vi "rs3 set device option2.vi"(8 "error in (no error)":errorcluster, 9 "value":sgl, 10 "RS Option":u16(ring) items=["    RS2_OPTION_BACKLIGHT_COMPENSATION                     , /**< Enable / disable color backlight compensation*/", "    RS2_OPTION_BRIGHTNESS                                 , /**< Color image brightness*/", "    RS2_OPTION_CONTRAST                                   , /**< Color image contrast*/", "    RS2_OPTION_EXPOSURE                                   , /**< Controls exposure time of color camera. Setting any value will disable auto exposure*/", "    RS2_OPTION_GAIN                                       , /**< Color image gain*/", "    RS2_OPTION_GAMMA                                      , /**< Color image gamma setting*/", "    RS2_OPTION_HUE                                        , /**< Color image hue*/", "    RS2_OPTION_SATURATION                                 , /**< Color image saturation setting*/", "    RS2_OPTION_SHARPNESS                                  , /**< Color image sharpness setting*/", "    RS2_OPTION_WHITE_BALANCE                              , /**< Controls white balance of color image. Setting any value will disable auto white balance*/", "    RS2_OPTION_ENABLE_AUTO_EXPOSURE                       , /**< Enable / disable color image auto-exposure*/", "    RS2_OPTION_ENABLE_AUTO_WHITE_BALANCE                  , /**< Enable / disable color image auto-white-balance*/", "    RS2_OPTION_VISUAL_PRESET                              , /**< Provide access to several recommend sets of option presets for the depth camera */", "    RS2_OPTION_LASER_POWER                                , /**< Power of the F200 / SR300 projector, with 0 meaning projector off*/", "    RS2_OPTION_ACCURACY                                   , /**< Set the number of patterns projected per frame. The higher the accuracy value the more patterns projected. Increasing the number of patterns help to achieve better accuracy. Note that this c", "    RS2_OPTION_MOTION_RANGE                               , /**< Motion vs. Range trade-off, with lower values allowing for better motion sensitivity and higher values allowing for better depth range*/", "    RS2_OPTION_FILTER_OPTION                              , /**< Set the filter to apply to each depth frame. Each one of the filter is optimized per the application requirements*/", "    RS2_OPTION_CONFIDENCE_THRESHOLD                       , /**< The confidence level threshold used by the Depth algorithm pipe to set whether a pixel will get a valid range or will be marked with invalid range*/", "    RS2_OPTION_EMITTER_ENABLED                            , /**< Laser Emitter enabled */", "    RS2_OPTION_FRAMES_QUEUE_SIZE                          , /**< Number of frames the user is allowed to keep per stream. Trying to hold-on to more frames will cause frame-drops.*/", "    RS2_OPTION_TOTAL_FRAME_DROPS                          , /**< Total number of detected frame drops from all streams */", "    RS2_OPTION_AUTO_EXPOSURE_MODE                         , /**< Auto-Exposure modes: Static, Anti-Flicker and Hybrid */", "    RS2_OPTION_AUTO_EXPOSURE_ANTIFLICKER_RATE             , /**< Auto-Exposure anti-flicker rate, can be 50 or 60 Hz */", "    RS2_OPTION_ASIC_TEMPERATURE                           , /**< Current Asic Temperature */", "    RS2_OPTION_ERROR_POLLING_ENABLED                      , /**< disable error handling */", "    RS2_OPTION_PROJECTOR_TEMPERATURE                      , /**< Current Projector Temperature */", "    RS2_OPTION_OUTPUT_TRIGGER_ENABLED                     , /**< Enable / disable trigger to be outputed from the camera to any external device on every depth frame */", "    RS2_OPTION_MOTION_MODULE_TEMPERATURE                  , /**< Current Motion-Module Temperature */", "    RS2_OPTION_DEPTH_UNITS                                , /**< Number of meters represented by a single depth unit */", "    RS2_OPTION_ENABLE_MOTION_CORRECTION                   , /**< Enable/Disable automatic correction of the motion data */", "    RS2_OPTION_COUNT                                      , /**< Number of enumeration values. Not a valid input: intended to be used in for-loops. */"], 11 "sensor in":u64) -> (0 "error out":errorcluster, 1 "error":u64, 3 "sensor out":u64)   [LabVIEW 2017, in "libRealSense3.lvlib"]
doc: "Sets the value of a specific device option\n \nInput:\noption the option whose value to set\nvalue the desired value to set\n \nOutput:\nerror if non-null, receives any error that occurs during this call, otherwise, errors are ignored"
uses:
  libRealSense3.lvlib
  realsense2.dll
panel:
  # "RS2_OPTION_BACKLIGHT_COMPENSATION                     , /**< Enable / disable color backlight compensation*/\n    RS2_OPTION_BRIGHTNESS                                 , /**< Color image brightness*/\n    RS2_OPTION_CONTRAST                                   , /**< Color image contrast*/\n    RS2_OPTION_EXPOSURE                                   , /**< Controls exposure time of color camera. Setting any value will disable auto exposure*/\n    RS2_OPTION_GAIN                                       , /**< Color image gain*/\n    RS2_OPTION_GAMMA                                      , /**< Color image gamma setting*/\n    RS2_OPTION_HUE                                        , /**< Color image hue*/\n    RS2_OPTION_SATURATION                                 , /**< Color image saturation setting*/\n    RS2_OPTION_SHARPNESS                                  , /**< Color image sharpness setting*/\n    RS2_OPTION_WHITE_BALANCE                              , /**< Controls white balance of color image. Setting any value will disable auto white balance*/\n    RS2_OPTION_ENABLE_AUTO_EXPOSURE                       , /**< Enable / disable color image auto-exposure*/\n    RS2_OPTION_ENABLE_AUTO_WHITE_BALANCE                  , /**< Enable / disable color image auto-white-balance*/\n    RS2_OPTION_VISUAL_PRESET                              , /**< Provide access to several recommend sets of option presets for the depth camera */\n    RS2_OPTION_LASER_POWER                                , /**< Power of the F200 / SR300 projector, with 0 meaning projector off*/\n    RS2_OPTION_ACCURACY                                   , /**< Set the number of patterns projected per frame. The higher the accuracy value the more patterns projected. Increasing the number of patterns help to achieve better accuracy. Note that this control is affecting the Depth FPS */\n    RS2_OPTION_MOTION_RANGE                               , /**< Motion vs. Range trade-off, with lower values allowing for better motion sensitivity and higher values allowing for better depth range*/\n    RS2_OPTION_FILTER_OPTION                              , /**< Set the filter to apply to each depth frame. Each one of the filter is optimized per the application requirements*/\n    RS2_OPTION_CONFIDENCE_THRESHOLD                       , /**< The confidence level threshold used by the Depth algorithm pipe to set whether a pixel will get a valid range or will be marked with invalid range*/\n    RS2_OPTION_EMITTER_ENABLED                            , /**< Laser Emitter enabled */\n    RS2_OPTION_FRAMES_QUEUE_SIZE                          , /**< Number of frames the user is allowed to keep per stream. Trying to hold-on to more frames will cause frame-drops.*/\n    RS2_OPTION_TOTAL_FRAME_DROPS                          , /**< Total number of detected frame drops from all streams */\n    RS2_OPTION_AUTO_EXPOSURE_MODE                         , /**< Auto-Exposure modes: Static, Anti-Flicker and Hybrid */\n    RS2_OPTION_AUTO_EXPOSURE_ANTIFLICKER_RATE             , /**< Auto-Exposure anti-flicker rate, can be 50 or 60 Hz */\n    RS2_OPTION_ASIC_TEMPERATURE                           , /**< Current Asic Temperature */\n    RS2_OPTION_ERROR_POLLING_ENABLED                      , /**< disable error handling */\n    RS2_OPTION_PROJECTOR_TEMPERATURE                      , /**< Current Projector Temperature */\n    RS2_OPTION_OUTPUT_TRIGGER_ENABLED                     , /**< Enable / disable trigger to be outputed from the camera to any external device on every depth frame */\n    RS2_OPTION_MOTION_MODULE_TEMPERATURE                  , /**< Current Motion-Module Temperature */\n    RS2_OPTION_DEPTH_UNITS                                , /**< Number of meters represented by a single depth unit */\n    RS2_OPTION_ENABLE_MOTION_CORRECTION                   , /**< Enable/Disable automatic correction of the motion data */\n    RS2_OPTION_COUNT"
  # "RS3 Set Device Options2"
  # "(C) 2016 Intel Corp.,  AGJ"
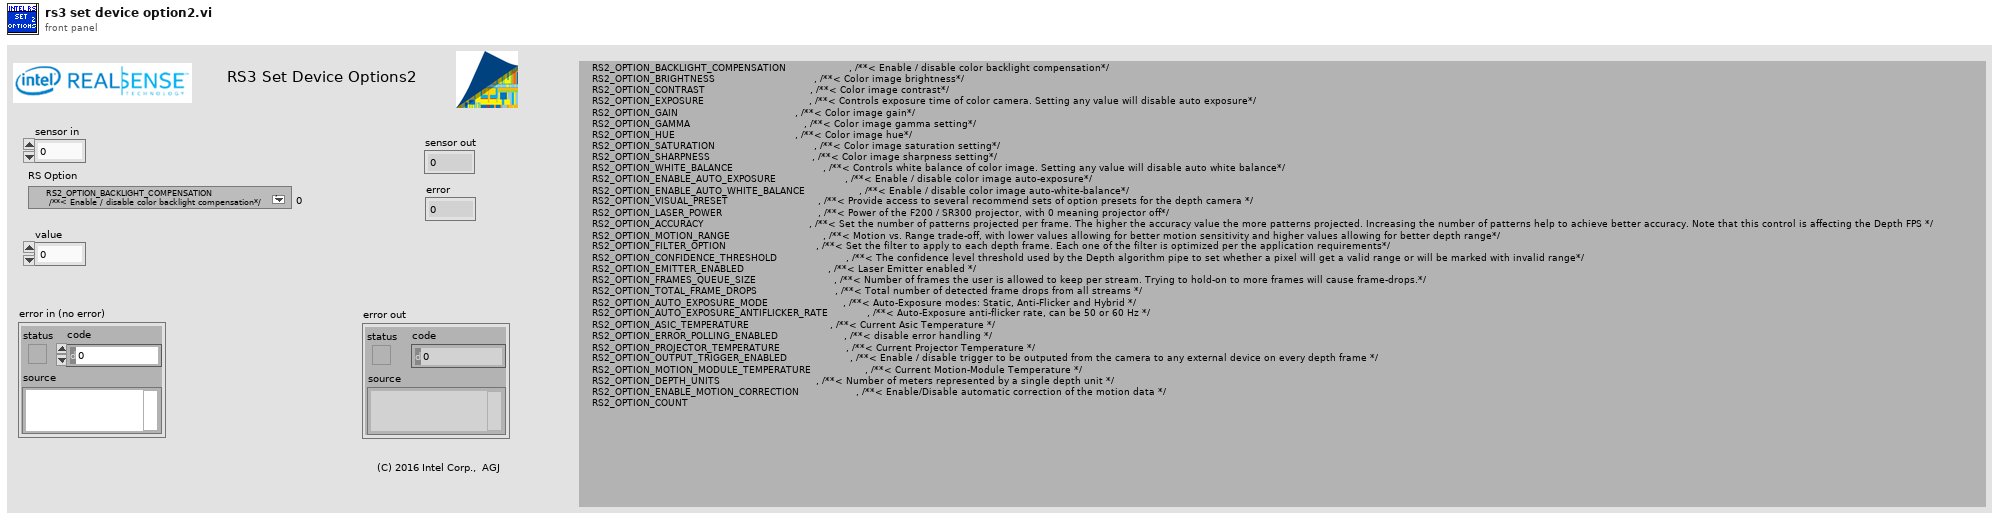
[diagram p1: front panel]
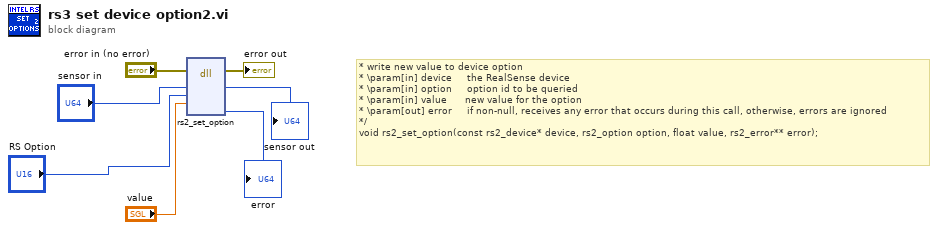
[diagram p0: block diagram]
diagram:
  # "* write new value to device option\n* \\param[in] device     the RealSense device\n* \\param[in] option     option id to be queried\n* \\param[in] value      new value for the option\n* \\param[out] error     if non-null, receives any error that occurs during this call, otherwise, errors are ignored\n*/\nvoid rs2_set_option(const rs2_device* device, rs2_option option, float value, rs2_error** error);"
  n1 = dll-call lib="C:/Users/agrunnet/Documents/libRealSense6/realsense2.dll" fn="rs2_set_option"(error in="error in (no error)", "device"="sensor in", "option"="RS Option", "value"="value") -> (error out=→"error out":errorcluster, "device"=→"sensor out":u64, "error"=→"error":u64)  [unwired: 6 in, 1 out]
